vi "Write CSV_Channel info.vi"(4 "MASTER in":T1 {"Image data"."Color Palette" items=["Grayscale U8", "False Color", "Overexposed"]; "Image data"."Exposure time [us]" format="%#_10g"; "Queue"."Initial time [s]" format="%_19f"; "Queue"."Raw data [V]\n(all samples)" format="%0.2f"; "Queue"."Timestamp [s]" format="%_19f"}) -> (1 "MASTER out":T1 {"Image data"."Color Palette" items=["Grayscale U8", "False Color", "Overexposed"]; "Image data"."Exposure time [us]" format="%#_10g"; "Queue"."Initial time [s]" format="%_19f"; "Queue"."Raw data [V]\n(all samples)" format="%0.2f"; "Queue"."Timestamp [s]" format="%_19f"})   [LabVIEW 2020]
uses:
  MASTER.ctl
  Constants.ctl
  QBundle.ctl
  Queue.ctl
  Image data.ctl
  <vilib>/userdefined/High Color/IMAQdx.ctl
  <vilib>/vision/Image Controls.llb/IMAQ Image.ctl
  Image QBundle.ctl
  <vilib>/Utility/file.llb/Write Delimited Spreadsheet (string).vi
panel:
  # "Description:\nWrites channel names, AS numbers, scale, and offset to separate .csv file in the same folder as data file."
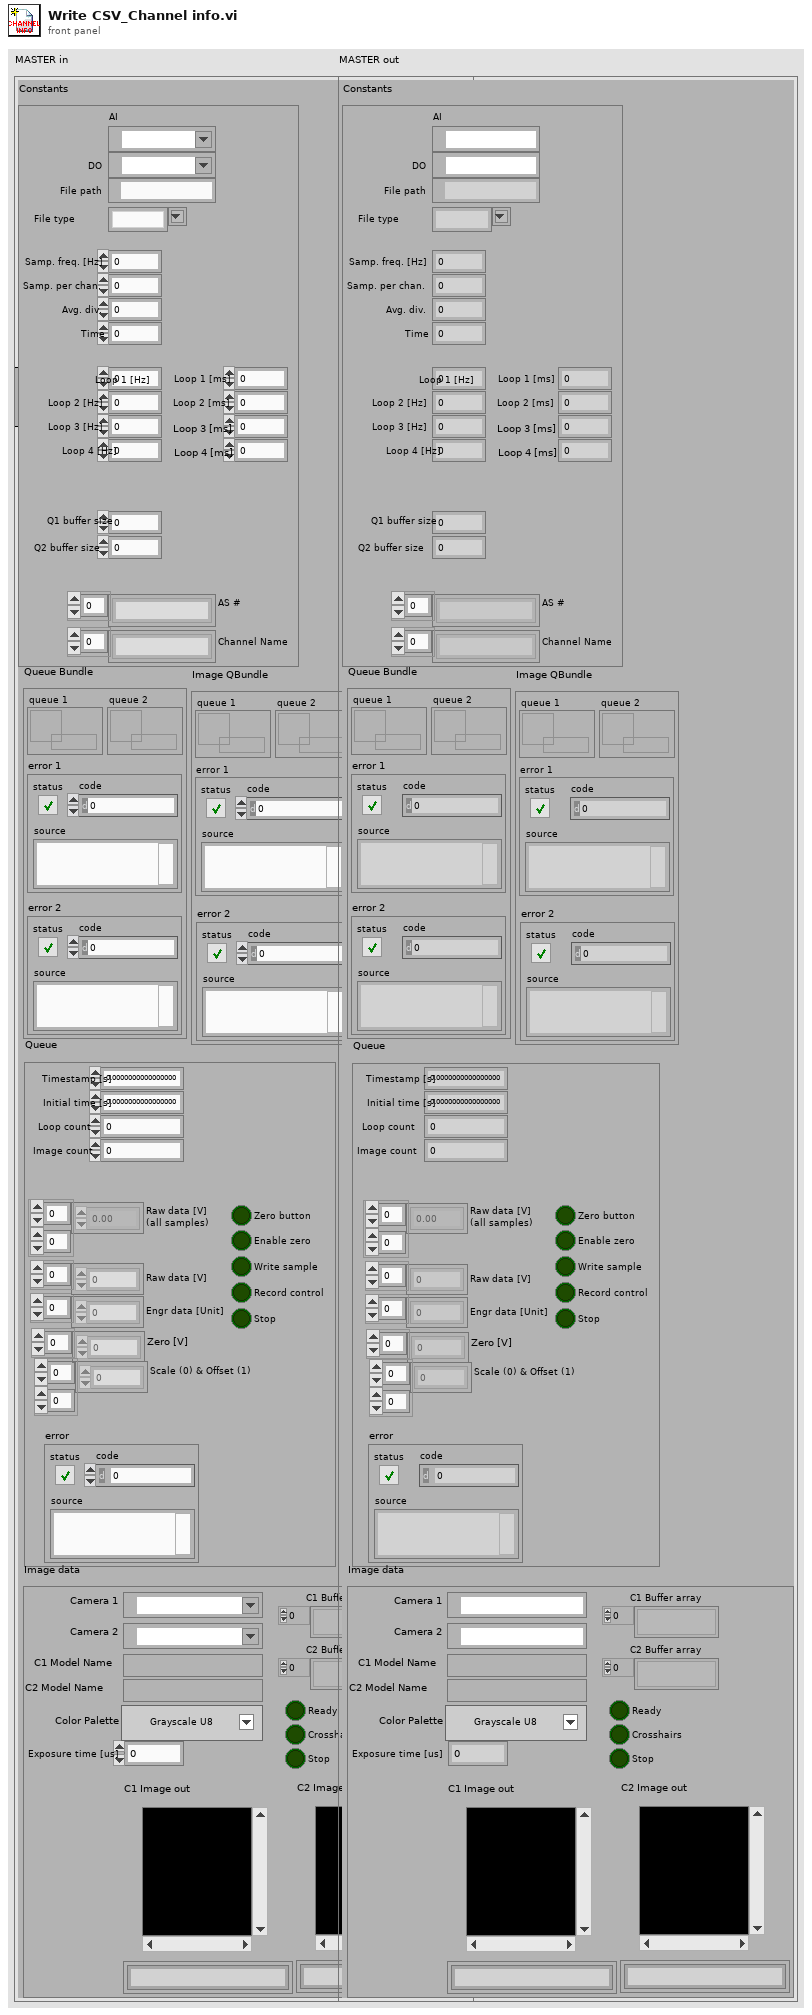
[diagram p1: front panel]
types:
  T1 = typedef "MASTER.ctl" = cluster{"Constants":T2, "Queue Bundle":T3, "Queue":T4, "Image data":T5, "Image QBundle ":T8}
  T2 = typedef "Constants.ctl" = cluster{"Time":u16, "Samp. freq. [Hz]":dbl, "Samp. per chan.":i32, "Avg. div.":i32, "File path":path, "AI":refnum<k21>, "Loop 1 [Hz]":dbl, "Loop 2 [Hz]":dbl, "Loop 3 [Hz]":dbl, "Loop 1 [ms]":dbl, "Loop 2 [ms]":dbl, "Loop 3 [ms]":dbl, "Q1 buffer size":i32, "Q2 buffer size":i32, "File type":string, "Loop 4 [Hz]":dbl, "Loop 4 [ms]":dbl, "Channel Name":string[], "AS #":string[], "DO":refnum<k21>}
  T3 = typedef "QBundle.ctl" = cluster{"queue 1":refnum<queue>, "error 1":errorcluster, "queue 2":refnum<queue>, "error 2":errorcluster}
  T4 = typedef "Queue.ctl" = cluster{"Enable zero":bool, "Engr data [Unit]":dbl[], "Zero button":bool, "Zero [V]":dbl[], "Timestamp [s]":dbl, "Write sample":bool, "Record control":bool, "Stop":bool, "error":errorcluster, "Raw data [V]\n(all samples)":dbl[][], "Raw data [V]":dbl[], "Loop count":i64, "Initial time [s]":dbl, "Scale (0) & Offset (1)":dbl[][], "Image count":dbl}
  T5 = typedef "Image data.ctl" = cluster{"Camera 1":T6, "Camera 2":T6, "C1 Image out ":T7, "C2 Image out":T7, "C1 Model Name":string, "C2 Model Name":string, "Exposure time [us]":dbl, "Color Palette":u16, "C1 Buffer array":T7[], "Ready":bool, "C2 Buffer array":T7[], "Crosshairs":bool, "Stop":bool}
  T6 = typedef "IMAQdx.ctl" = refnum<k21>
  T7 = typedef "IMAQ Image.ctl" = refnum<image>
  T8 = typedef "Image QBundle.ctl" = cluster{"queue 1":refnum<queue>, "error 1":errorcluster, "queue 2":refnum<queue>, "error 2":errorcluster}
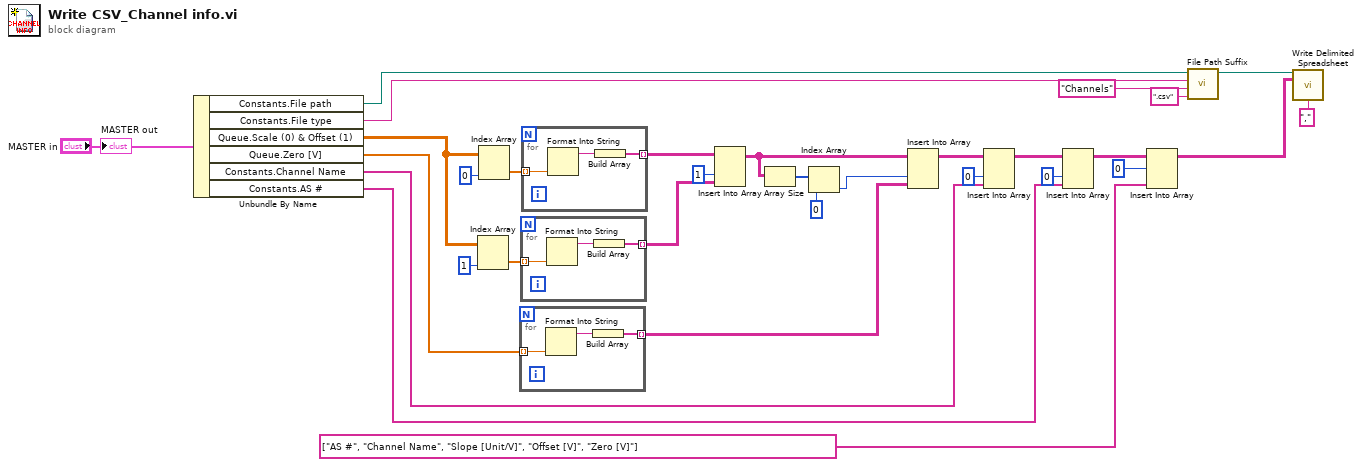
[diagram p0: block diagram]
diagram:
  n1 = Unbundle By Name("MASTER in") -> ("Constants.File path"=w2:path, "Constants.File type"=w1:string, "Queue.Scale (0) & Offset (1)"=w7:dbl[][], "Queue.Zero [V]"=w6:dbl[], "Constants.Channel Name"=w5:string[], "Constants.AS #"=w4:string[])
  n2 = Index Array(array=w7, index (col)=1 ("disabled index (col)")) -> (element=w28:dbl[])  [unwired: 1 in]
  n3 = Index Array(array=w7, index (col)=0 ("disabled index (col)")) -> (element=w30:dbl[])  [unwired: 1 in]
  n4 = for {
    tunnel: w6 -> [w34] mode=indexing
    tunnel: [w32] -> w13 mode=indexing
    n5 = Format Into String(w34) -> (resulting string=w33:string)  [unwired: 3 in, 1 out]
    n6 = Build Array(w33) -> (w32:string[])
  }
  n7 = for {
    tunnel: w28 -> [w37] mode=indexing
    tunnel: [w35] -> w25 mode=indexing
    n8 = Format Into String(w37) -> (resulting string=w36:string)  [unwired: 3 in, 1 out]
    n9 = Build Array(w36) -> (w35:string[])
  }
  n10 = for {
    tunnel: w30 -> [w40] mode=indexing
    tunnel: [w38] -> w26 mode=indexing
    n11 = Format Into String(w40) -> (resulting string=w39:string)  [unwired: 3 in, 1 out]
    n12 = Build Array(w39) -> (w38:string[])
  }
  n13 = Insert Into Array(array=w26, index (col)=1 ("disabled index (col)"), new element=w25) -> (w12:string[][])  [unwired: 1 in]
  n14 = Array Size(array=w12) -> (size(s)=w11:i32[])
  n15 = Index Array(array=w11, index=0) -> (element=w9:i32)
  n16 = Insert Into Array(array=w12, index (col)=w9, new element=w13) -> (w20:string[][])  [unwired: 1 in]
  n17 = Insert Into Array(array=w20, index (col)=0 ("disabled index (col)"), new element=w5) -> (w15:string[][])  [unwired: 1 in]
  n18 = Insert Into Array(array=w15, index (col)=0 ("disabled index (col)"), new element=w4) -> (w14:string[][])  [unwired: 1 in]
  n19 = Insert Into Array(array=w14, index (row)=0, new element=string[] ["AS #", "Channel Name", "Slope [Unit/V]", "Offset [V]", "Zero [V]"] ("array")) -> (w21:string[][])  [unwired: 1 in]
  n20 = call "File Path Suffix.vi"("Data file type"=".csv" ("File type"), "Suffix string"="Channels" ("new element/subarray"), "File type"=w1, "File path"=w2) -> ("New file path"=w17:path)  [unwired: 7 in]
  n21 = call-poly <vilib>:"Write Delimited Spreadsheet.vi"("file path (dialog if empty)"=w17, "2D data"=w21, "delimiter (\\t)"="," ("delimiter (\\t)")) -> ()  [unwired: 11 in, 2 out]
  "MASTER out" <- "MASTER in"
